vi "Get camera FOVs.vi"(10 "Camera Type":T1(ring)) -> (1 "Camera view angles":dbl[](array[numeric])=[51.7, 49.4, 64.0, 52.0, 41.0], 3 "FOV":dbl=41.0)   [LabVIEW 2015]
doc: "Return the view angle for common FRC cameras. This is useful for calculating distances to objects in captured images."
panel:
  in  "Camera view angles":dbl[](array[numeric])=[51.7, 49.4, 64.0, 52.0, 60.0]
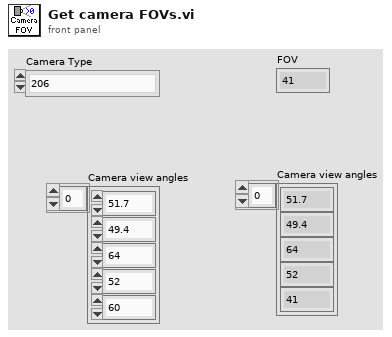
[diagram p1: front panel]
types:
  T1 = enum16{"206", "1011", "1013", "MS HD3000 square", "MS HD3000 640x480"}
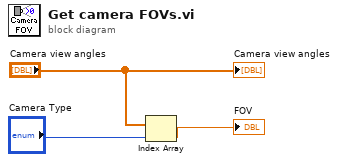
[diagram p0: block diagram]
diagram:
  n1 = Index Array(array="Camera view angles", index="Camera Type") -> (element=→"FOV":dbl)
  "Camera view angles" <- "Camera view angles"
